vi "Autonomous Independent.vi"() -> ()   [LabVIEW 2013]
doc: "This VI is called when autonomous begins, and will automatically be terminated when autonomous ends. You can carry out timed or sensor driven robot movement independently without needing to return to the caller."
uses:
  Robot Global Data.vi
  DoubleSolenoidAction.ctl
  OneBall.ctl
  TankDriveAction.ctl
  ShooterAction.ctl
  TwoBall.ctl
  CollectorAction.ctl
  RollerAction.ctl
panel:
  in  "Error in 2":errorcluster
  out "Error out 2":errorcluster
  in  "Error in":errorcluster
  out "Error out":errorcluster
  # "Be sure to right-click and choose Data Operations>>Make Current Value default if you want to save the array values with the VI"
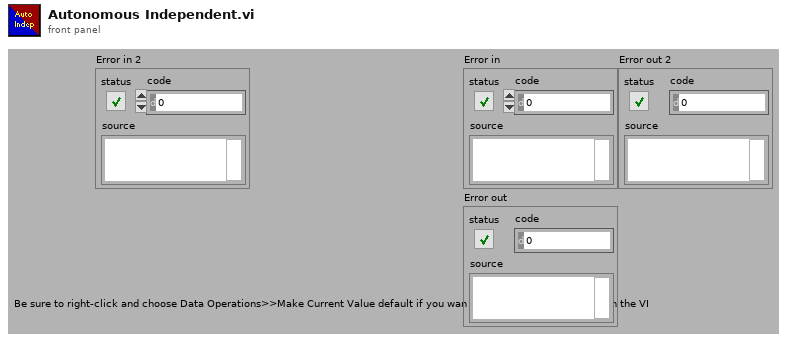
[diagram p1: front panel]
types:
  T1 = typedef "TwoBall.ctl" = enum16{"Init", "Lower Arm", "Spin Roller", "Clapper", "RaiseArmSlightly", "Drive", "Shoot1", "RaiseArmUp", "Shoot2", "Stop"}
  T2 = typedef "OneBall.ctl" = enum16{"Init", "Drive", "Shoot", "CheckGoal", "Stop"}
  T3 = typedef "DoubleSolenoidAction.ctl" = enum16{"Init", "Out", "In", "Middle"}
  T4 = typedef "TankDriveAction.ctl" = enum16{"Init", "LinearDrive", "SetValue", "Disable"}
  T5 = typedef "ShooterAction.ctl" = enum16{"Init", "Shoot"}
  T6 = typedef "WPI_SolenoidDevRef.ctl" = cluster{"DevStatus":errorcluster, "Solenoid Module":T7, "Forward Solenoid Channel":T8, "Reverse Solenoid Channel":T8}
  T7 = typedef "FPGA_TypedefSolenoidModule.ctl" = enum16{"Solenoid Module 1", "Solenoid Module 2"}
  T8 = typedef "WPI_SolenoidChannel.ctl" = enum8{"Solenoid 1", "Solenoid 2", "Solenoid 3", "Solenoid 4", "Solenoid 5", "Solenoid 6", "Solenoid 7", "Solenoid 8", "Invalid"}
  T9 = typedef "CollectorAction.ctl" = enum16{"Init", "Raise", "Lower", "Stop", "GetStatus"}
  T10 = typedef "RollerAction.ctl" = enum16{"Init", "Off", "Forward", "Reverse"}
  T11 = typedef "WPI_RelayDevRef.ctl" = cluster{"DevStatus":errorcluster, "Relay Channel":T12, "Digital Module":T13, "Relay Direction":T14}
  T12 = typedef "FPGA_DIORelayChannel.ctl" = enum8{"Relay 1", "Relay 2", "Relay 3", "Relay 4", "Relay 5", "Relay 6", "Relay 7", "Relay 8", "Invalid"}
  T13 = typedef "FPGA_TypedefDigitalModule.ctl" = enum16{"Digital Module 1", "Digital Module 2"}
  T14 = typedef "WPI_RelayDirection.ctl" = enum16{"Both directions", "Forward only", "Reverse only"}
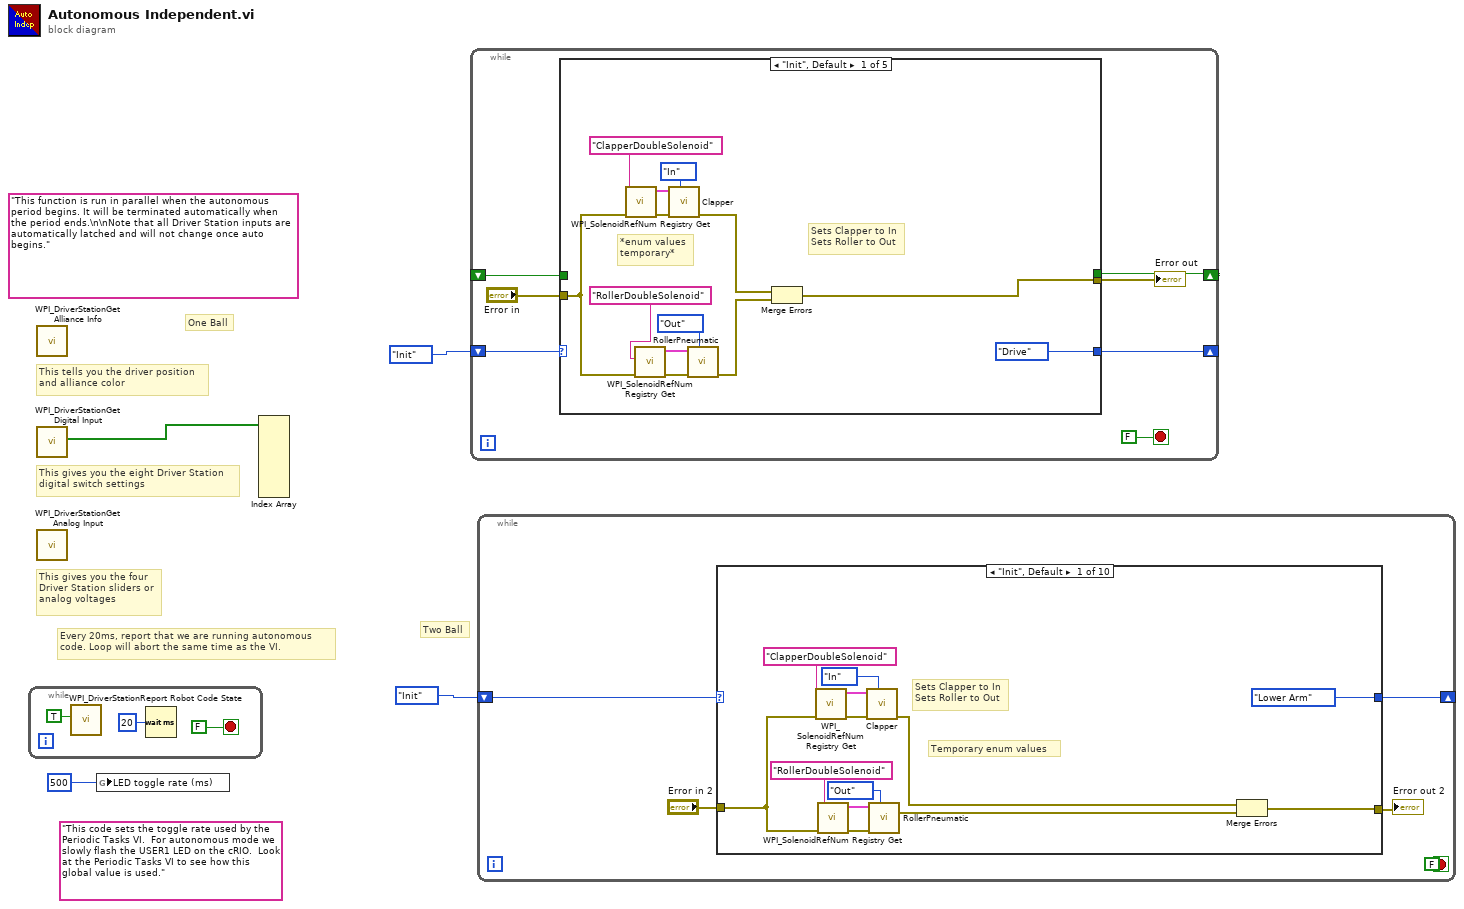
[diagram p0: block diagram]
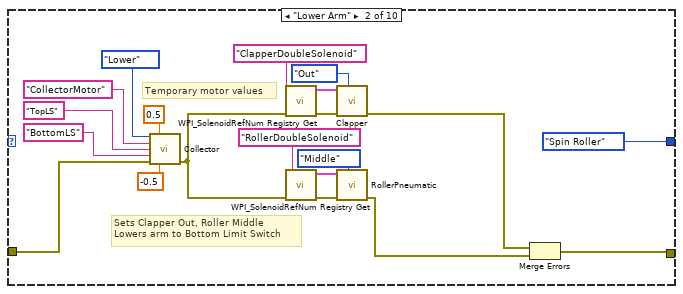
[diagram p2: hidden frame]
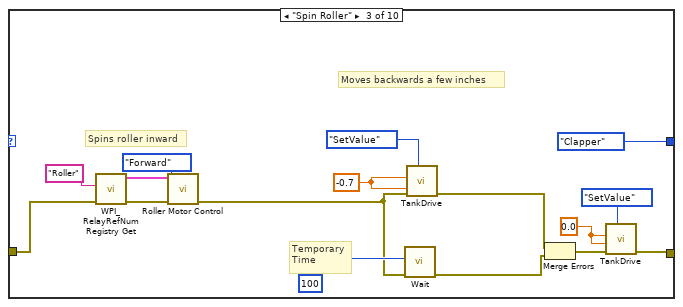
[diagram p3: hidden frame]
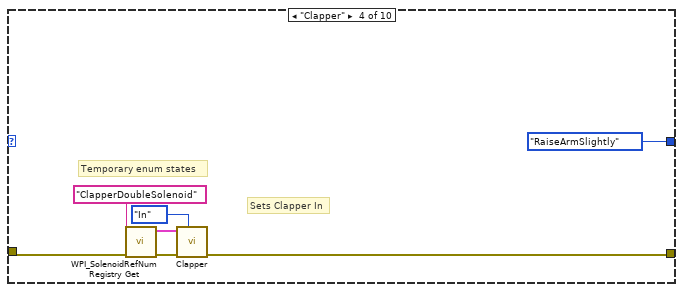
[diagram p4: hidden frame]
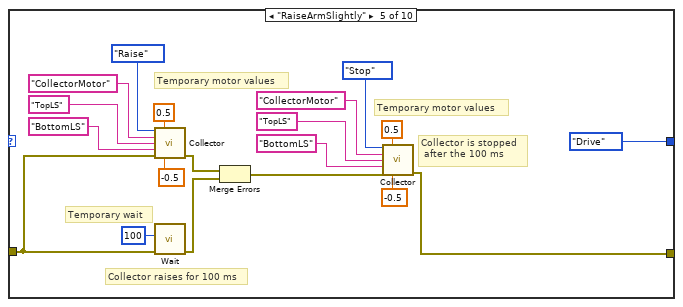
[diagram p5: hidden frame]
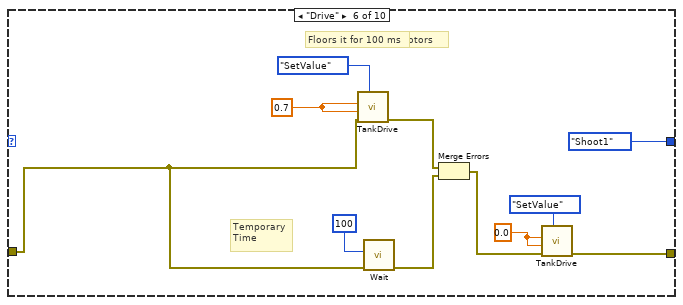
[diagram p6: hidden frame]
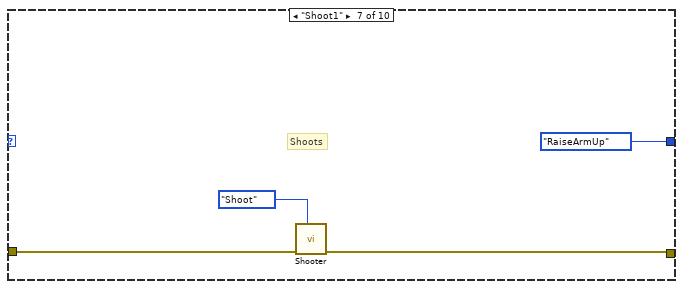
[diagram p7: hidden frame]
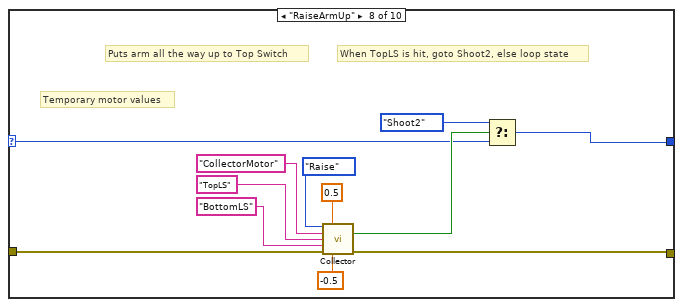
[diagram p8: hidden frame]
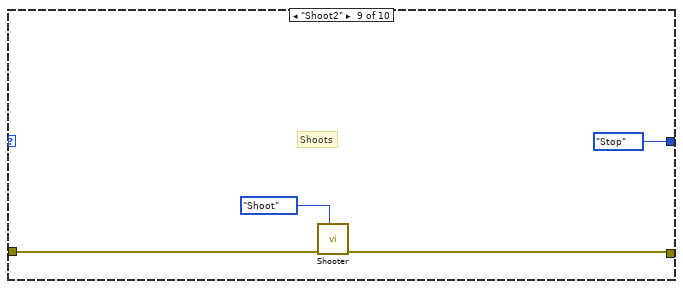
[diagram p9: hidden frame]
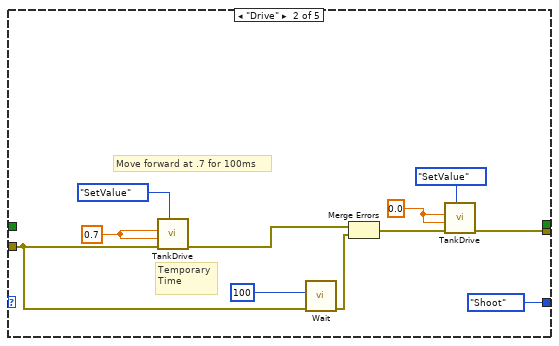
[diagram p11: hidden frame]
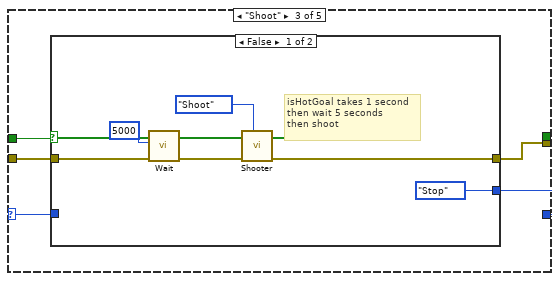
[diagram p12: hidden frame]
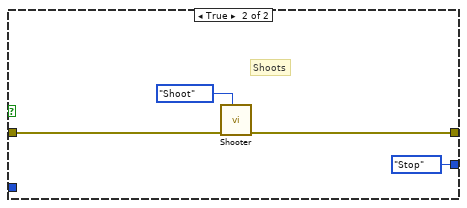
[diagram p13: hidden frame]
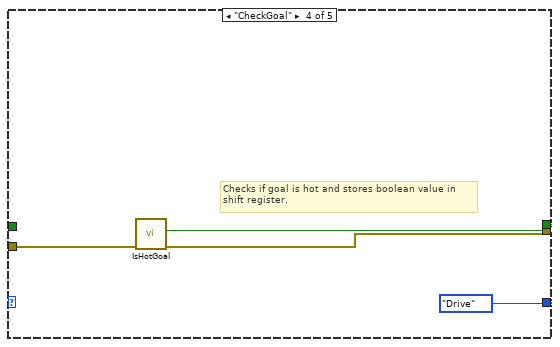
[diagram p14: hidden frame]
diagram:
  (unwired) "This code sets the toggle rate used by the Periodic Tasks VI.  For autonomous mode we slowly flash the USER1 LED on the cRIO.  Look at the Periodic Tasks VI to see how this global value is used."
  (unwired) "This function is run in parallel when the autonomous period begins. It will be terminated automatically when the period ends.\n\nNote that all Driver Station inputs are automatically latched and will not change once auto begins."
  # "Two Ball"
  # "One Ball"
  # "Every 20ms, report that we are running autonomous\ncode. Loop will abort the same time as the VI."
  # "This tells you the driver position\nand alliance color"
  # "This gives you the eight Driver Station\ndigital switch settings"
  # "This gives you the four\nDriver Station sliders or\nanalog voltages"
  n1 = while {
    stop <- FALSE stop-if-true
    n2 = call <vilib>:"WPI_DriverStationReport Robot Code State.vi"("Autonomous"=TRUE) -> ()  [unwired: 10 in, 1 out]
    n3 = Wait (ms)(milliseconds to wait=u32 20) -> ()  [unwired: 1 out]
  }
  n4 = call <vilib>:"WPI_DriverStationGet Alliance Info.vi"() -> ()  [unwired: 12 out]
  n5 = call <vilib>:"WPI_DriverStationGet Digital Input.vi"() -> ("Driver Station Digital Input (1-8)"=w4:bool[])  [unwired: 11 out]
  n6 = call <vilib>:"WPI_DriverStationGet Analog Input.vi"() -> ()  [unwired: 12 out]
  n7 = global write "Robot Global Data.vi" "LED toggle rate (ms)"(u32 500 ("LED ms toggle rate")) -> ()
  n8 = Index Array(array=w4) -> ()  [unwired: 8 in, 8 out]
  n9 = while {
    shift-right: [w11] -> _
    shift-left: OneBall."Init" -> [w10]
    shift-right: [w9] -> _
    shift-left: _ -> [w8]
    stop <- FALSE stop-if-true
    n10 = case shown="\"Init\", Default" w10 {
      selector: w10 -> [_ _ w42 _ _]
      tunnel: [w25 w30 w39 w56 w58] -> w14
      tunnel: "Error in" -> [w17 w33 w40 w57 w58]
      tunnel: [OneBall."Drive" OneBall."Shoot" w43 OneBall."Drive" _] -> w11
      tunnel: [_ _ _ w54 _] -> w9
      tunnel: w8 -> [_ _ w41 _ _]
      frame "Init", Default {
        # "Sets Clapper to In\nSets Roller to Out"
        # "*enum values\ntemporary*"
        n11 = call <vilib>:"WPI_SolenoidRefNum Registry Get.vi"("error in (no error)"=w17, "refnum name"="ClapperDoubleSolenoid") -> ("error out"=w23:errorcluster, "SolenoidDevRef"=w26:T6)  [unwired: 8 in]
        n12 = call <vilib>:"WPI_SolenoidRefNum Registry Get.vi"("error in (no error)"=w17, "refnum name"="RollerDoubleSolenoid") -> ("error out"=w19:errorcluster, "SolenoidDevRef"=w20:T6)  [unwired: 8 in]
        n13 = call "Clapper.vi"("State"=DoubleSolenoidAction."In", "Error in"=w23, "SolenoidDevRef"=w26) -> ("Error out"=w24:errorcluster)  [unwired: 8 in]
        n14 = call "RollerPneumatic.vi"("State"=DoubleSolenoidAction."Out", "Error in"=w19, "SolenoidDevRef"=w20) -> ("Error out"=w15:errorcluster)  [unwired: 8 in]
        n15 = Merge Errors(w24, w15) -> (w25:errorcluster)
      }
      frame "Drive" {
        w28 = 0.0
        w34 = 0.7 ("RightDesired")
        # "Move forward at .7 for 100ms"
        # "Temporary\nTime"
        n16 = call "TankDrive.vi"("DriveAction"=TankDriveAction."SetValue", "error in (no error)"=w33, "RightDesired"=w34, "LeftDesired"=w34) -> ("error out"=w32:errorcluster)  [unwired: 7 in]
        n17 = call "Wait.vi"("error in"=w33, "milliseconds to wait"=u32 100) -> ("error out"=w35:errorcluster)  [unwired: 9 in]
        n18 = Merge Errors(w32, w35) -> (w38:errorcluster)
        n19 = call "TankDrive.vi"("DriveAction"=TankDriveAction."SetValue", "error in (no error)"=w38, "RightDesired"=w28, "LeftDesired"=w28) -> ("error out"=w30:errorcluster)  [unwired: 7 in]
      }
      frame "Shoot" {
        n20 = case shown="False" w41 {
          tunnel: w42 -> [_ _]
          tunnel: [OneBall."Stop" OneBall."Stop"] -> w43
          tunnel: w40 -> [w48 w52]
          tunnel: [w46 w51] -> w39
          frame False {
            # "isHotGoal takes 1 second\nthen wait 5 seconds\nthen shoot"
            n21 = call "Wait.vi"("error in"=w48, "milliseconds to wait"=u32 5000) -> ("error out"=w47:errorcluster)  [unwired: 9 in]
            n22 = call "Shooter.vi"("Action"=ShooterAction."Shoot", "error in"=w47) -> ("error out"=w46:errorcluster)  [unwired: 9 in]
          }
          frame True {
            # "Shoots"
            n23 = call "Shooter.vi"("Action"=ShooterAction."Shoot", "error in"=w52) -> ("error out"=w51:errorcluster)  [unwired: 9 in]
          }
        }
      }
      frame "CheckGoal" {
        # "Checks if goal is hot and stores boolean value in\nshift register."
        n24 = call "IsHotGoal.vi"("error in"=w57) -> ("error out"=w56:errorcluster, "Hot/Not"=w54:bool)  [unwired: 9 in]
      }
      frame "Stop" {
        # "Stop?"
      }
    }
    "Error out" <- w14
  }
  n25 = while {
    shift-right: [w61] -> _
    shift-left: TwoBall."Init" ("Enum") -> [w62]
    stop <- FALSE stop-if-true
    n26 = case shown="\"Init\", Default" w62 {
      selector: w62 -> [_ _ _ _ _ _ _ w154 _ _]
      tunnel: [TwoBall."Lower Arm" ("Enum") TwoBall."Spin Roller" ("Enum") TwoBall."Clapper" ("Enum") TwoBall."RaiseArmSlightly" ("Enum") TwoBall."Drive" ("Enum") TwoBall."Shoot1" ("Enum") TwoBall."RaiseArmUp" ("Enum") w157 TwoBall."Stop" ("Enum") _] -> w61
      tunnel: "Error in 2" -> [w67 w95 w108 w115 w133 w144 w152 w160 w168 w170]
      tunnel: [w64 w82 w99 w114 w121 w141 w151 w159 w167 w170] -> w59
      frame "Init", Default {
        # "Sets Clapper to In\nSets Roller to Out"
        # "Temporary enum values"
        n27 = call <vilib>:"WPI_SolenoidRefNum Registry Get.vi"("error in (no error)"=w67, "refnum name"="ClapperDoubleSolenoid") -> ("error out"=w74:errorcluster, "SolenoidDevRef"=w75:T6)  [unwired: 8 in]
        n28 = call <vilib>:"WPI_SolenoidRefNum Registry Get.vi"("error in (no error)"=w67, "refnum name"="RollerDoubleSolenoid") -> ("error out"=w72:errorcluster, "SolenoidDevRef"=w70:T6)  [unwired: 8 in]
        n29 = call "Clapper.vi"("State"=DoubleSolenoidAction."In", "Error in"=w74, "SolenoidDevRef"=w75) -> ("Error out"=w66:errorcluster)  [unwired: 8 in]
        n30 = call "RollerPneumatic.vi"("State"=DoubleSolenoidAction."Out", "Error in"=w72, "SolenoidDevRef"=w70) -> ("Error out"=w65:errorcluster)  [unwired: 8 in]
        n31 = Merge Errors(w66, w65) -> (w64:errorcluster)
      }
      frame "Lower Arm" {
        # "Sets Clapper Out, Roller Middle\nLowers arm to Bottom Limit Switch"
        # "Temporary motor values"
        n32 = call "Collector.vi"("CollectorAction"=CollectorAction."Lower", "Raise"=0.5, "CollectorMotor"="CollectorMotor", "TopLS"="TopLS", "BottomLS"="BottomLS", "Error in"=w95, "Lower"=-0.5) -> ("Error out"=w83:errorcluster)  [unwired: 6 in, 2 out]
        n33 = call <vilib>:"WPI_SolenoidRefNum Registry Get.vi"("error in (no error)"=w83, "refnum name"="ClapperDoubleSolenoid") -> ("error out"=w86:errorcluster, "SolenoidDevRef"=w85:T6)  [unwired: 8 in]
        n34 = call <vilib>:"WPI_SolenoidRefNum Registry Get.vi"("error in (no error)"=w83, "refnum name"="RollerDoubleSolenoid") -> ("error out"=w88:errorcluster, "SolenoidDevRef"=w90:T6)  [unwired: 8 in]
        n35 = call "Clapper.vi"("State"=DoubleSolenoidAction."Out", "Error in"=w86, "SolenoidDevRef"=w85) -> ("Error out"=w81:errorcluster)  [unwired: 8 in]
        n36 = call "RollerPneumatic.vi"("State"=DoubleSolenoidAction."Middle", "Error in"=w88, "SolenoidDevRef"=w90) -> ("Error out"=w80:errorcluster)  [unwired: 8 in]
        n37 = Merge Errors(w81, w80) -> (w82:errorcluster)
      }
      frame "Spin Roller" {
        w97 = 0.0
        w104 = -0.7
        # "Spins roller inward"
        # "Moves backwards a few inches"
        # "Temporary\nTime"
        n38 = call <vilib>:"WPI_RelayRefNum Registry Get.vi"("error in (no error)"=w108, "refnum name"="Roller") -> ("error out"=w111:errorcluster, "RelayDevRef"=w112:T11)  [unwired: 8 in]
        n39 = call "Roller Motor Control.vi"("Error in"=w111, "RollerState"=RollerAction."Forward", "RelayDevRef"=w112) -> ("Error out"=w100:errorcluster)  [unwired: 8 in]
        n40 = call "Wait.vi"("error in"=w100, "milliseconds to wait"=u32 100) -> ("error out"=w101:errorcluster)  [unwired: 9 in]
        n41 = call "TankDrive.vi"("DriveAction"=TankDriveAction."SetValue", "error in (no error)"=w100, "RightDesired"=w104, "LeftDesired"=w104) -> ("error out"=w102:errorcluster)  [unwired: 7 in]
        n42 = Merge Errors(w102, w101) -> (w106:errorcluster)
        n43 = call "TankDrive.vi"("DriveAction"=TankDriveAction."SetValue", "error in (no error)"=w106, "RightDesired"=w97, "LeftDesired"=w97) -> ("error out"=w99:errorcluster)  [unwired: 7 in]
      }
      frame "Clapper" {
        # "Sets Clapper In"
        # "Temporary enum states"
        n44 = call <vilib>:"WPI_SolenoidRefNum Registry Get.vi"("error in (no error)"=w115, "refnum name"="ClapperDoubleSolenoid") -> ("error out"=w117:errorcluster, "SolenoidDevRef"=w118:T6)  [unwired: 8 in]
        n45 = call "Clapper.vi"("State"=DoubleSolenoidAction."In", "Error in"=w117, "SolenoidDevRef"=w118) -> ("Error out"=w114:errorcluster)  [unwired: 8 in]
      }
      frame "RaiseArmSlightly" {
        # "Collector is stopped\n after the 100 ms"
        # "Collector raises for 100 ms"
        # "Temporary motor values"
        # "Temporary motor values"
        # "Temporary wait"
        n46 = call "Collector.vi"("CollectorAction"=CollectorAction."Raise", "Raise"=0.5, "CollectorMotor"="CollectorMotor", "TopLS"="TopLS", "BottomLS"="BottomLS", "Error in"=w133, "Lower"=-0.5) -> ("Error out"=w130:errorcluster)  [unwired: 6 in, 2 out]
        n47 = call "Wait.vi"("error in"=w133, "milliseconds to wait"=u32 100) -> ("error out"=w129:errorcluster)  [unwired: 9 in]
        n48 = Merge Errors(w130, w129) -> (w125:errorcluster)
        n49 = call "Collector.vi"("CollectorAction"=CollectorAction."Stop", "Raise"=0.5, "CollectorMotor"="CollectorMotor", "TopLS"="TopLS", "BottomLS"="BottomLS", "Error in"=w125, "Lower"=-0.5) -> ("Error out"=w121:errorcluster)  [unwired: 6 in, 2 out]
      }
      frame "Drive" {
        w139 = 0.0
        w145 = 0.7 ("RightDesired")
        # "0.7 speed for both motors"
        # "Floors it for 100 ms"
        # "Temporary\nTime"
        n50 = call "TankDrive.vi"("DriveAction"=TankDriveAction."SetValue", "error in (no error)"=w144, "RightDesired"=w145, "LeftDesired"=w145) -> ("error out"=w143:errorcluster)  [unwired: 7 in]
        n51 = call "Wait.vi"("error in"=w144, "milliseconds to wait"=u32 100) -> ("error out"=w146:errorcluster)  [unwired: 9 in]
        n52 = Merge Errors(w143, w146) -> (w147:errorcluster)
        n53 = call "TankDrive.vi"("DriveAction"=TankDriveAction."SetValue", "error in (no error)"=w147, "RightDesired"=w139, "LeftDesired"=w139) -> ("error out"=w141:errorcluster)  [unwired: 7 in]
      }
      frame "Shoot1" {
        # "Shoots"
        n54 = call "Shooter.vi"("Action"=ShooterAction."Shoot", "error in"=w152) -> ("error out"=w151:errorcluster)  [unwired: 9 in]
      }
      frame "RaiseArmUp" {
        # "When TopLS is hit, goto Shoot2, else loop state"
        # "Puts arm all the way up to Top Switch"
        # "Temporary motor values"
        n55 = call "Collector.vi"("CollectorAction"=CollectorAction."Raise", "Raise"=0.5, "CollectorMotor"="CollectorMotor", "TopLS"="TopLS", "BottomLS"="BottomLS", "Error in"=w160, "Lower"=-0.5) -> ("Upper Triggered?"=w156:bool, "Error out"=w159:errorcluster)  [unwired: 6 in, 1 out]
        n56 = Select(t=TwoBall."Shoot2" ("Enum"), s=w156, f=w154) -> (s? t:f=w157:T1)
      }
      frame "Shoot2" {
        # "Shoots"
        n57 = call "Shooter.vi"("Action"=ShooterAction."Shoot", "error in"=w168) -> ("error out"=w167:errorcluster)  [unwired: 9 in]
      }
      frame "Stop" {
        # "Stop?"
      }
    }
    "Error out 2" <- w59
  }
